vi "Abort_HornScan_SUB_VI.vi"(4 "Response ID 1":u8=68, 6 "Operation Message Length 1":i32, 8 "Operation Message ID 1":i32=67, 9 "error in (no error)":errorcluster, 10 "Socket_IP_Address":u16, 11 "Socket_IP_Address":string) -> (0 "error out":errorcluster, 3 "connection ID":refnum<k5>, 5 "Pass":string="Horn Scan Success")   [LabVIEW 2017]
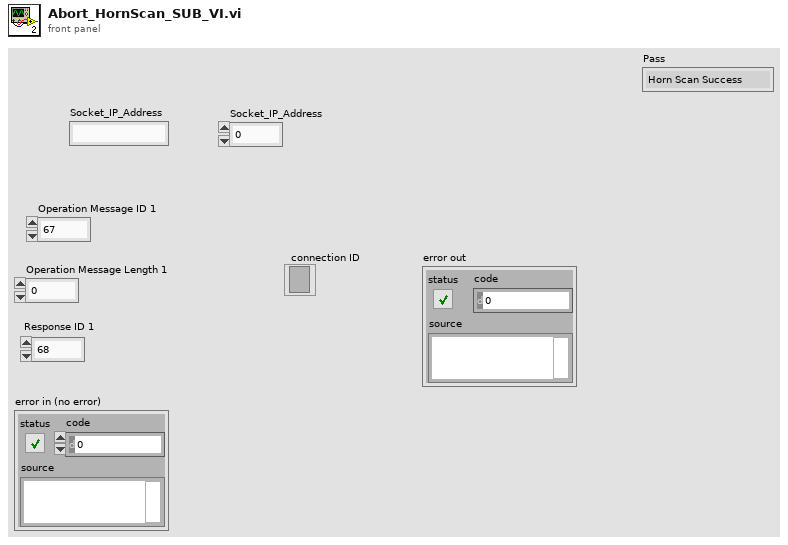
[diagram p1: front panel]
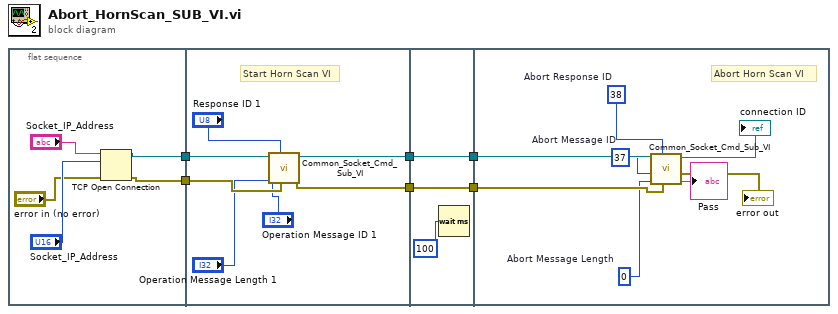
[diagram p0: block diagram]
diagram:
  n1 = flat-sequence {
    tunnel: [w8] -> w6
    tunnel: [w7] -> w5
    tunnel: w6 -> [w18]
    tunnel: w5 -> [w17]
    tunnel: [w13] -> w4
    tunnel: [w12] -> w2
    tunnel: w4 -> [w21]
    tunnel: [w21] -> w3
    tunnel: w2 -> [w20]
    tunnel: [w20] -> w1
    tunnel: w3 -> [w29]
    tunnel: w1 -> [w28]
    frame #0 {
      n2 = TCP Open Connection(address="Socket_IP_Address", remote port or service name="Socket_IP_Address", error in (no error)="error in (no error)") -> (connection ID=w8:refnum<k5>, error out=w7:errorcluster)  [unwired: 2 in]
    }
    frame #1 {
      # "Start Horn Scan VI"
      n3 = call "Common_Socket_Cmd_Sub_VI.vi"("Common Socket Error in"=w17, "Response ID 1"="Response ID 1", "Operation Message Length 1"="Operation Message Length 1", "Operation Message ID 1"="Operation Message ID 1", "connection ID"=w18) -> ("error out"=w12:errorcluster, "connection ID"=w13:refnum<k5>)  [unwired: 4 in, 1 out]
    }
    frame #2 {
      n4 = Wait (ms)(milliseconds to wait=u32 100) -> ()  [unwired: 1 out]
    }
    frame #3 {
      w26 = 0  # Abort Message Length
      w25 = 37  # Abort Message ID
      w27 = u8 38  # Abort Response ID
      # "Abort Horn Scan VI"
      n5 = call "Common_Socket_Cmd_Sub_VI.vi"("Common Socket Error in"=w28, "Response ID 1"=w27, "Operation Message Length 1"=w26, "Operation Message ID 1"=w25, "connection ID"=w29) -> ("Pass"=→"Pass":string, "error out"=→"error out":errorcluster, "connection ID"=→"connection ID":refnum<k5>)  [unwired: 4 in]
    }
  }
